vi "DatabaseHand_FindSubElement.vi"(8 "error in (no error)":errorcluster, 10 "name":string, 11 "Database RefNum in":T3) -> (0 "error out":errorcluster, 1 "index":i32, 2 "Database":T1, 3 "Database RefNum out":T3, 4 "object index":i32)   [LabVIEW 2016]
doc: "This VI finds the RefNum of an existing object with the input Name or creates a new object if the Name is not found or Name is unwired or an empty string.\nCopyright 2001 VI Engineering, Inc."
uses:
  DatabaseHand_RefNum.ctl
  DatabaseHand_Element.ctl
  DatabaseHan_DatabaseElement.ctl
  DatabaseHand_Function.ctl
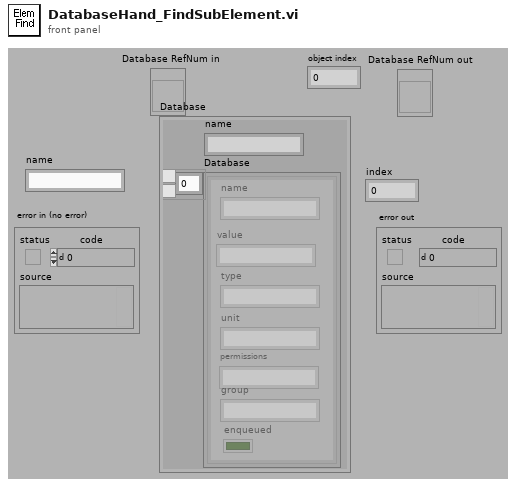
[diagram p1: front panel]
types:
  T1 = typedef "DatabaseHand_Element.ctl" = cluster{"name":string, "Database":T2[]}
  T2 = typedef "DatabaseHan_DatabaseElement.ctl" = cluster{"name":string, "value":string, "type":string, "unit":string, "permissions":string, "enqueued":bool, "group":string}
  T3 = typedef "DatabaseHand_RefNum.ctl" = refnum<vi>
  T4 = typedef "DatabaseHand_Function.ctl" = enum16{"Reset", "Register", "Get Data", "Set Data", "Unregister", "Test", "Get Objects", "Delete Data"}
  T5 = typedef "Database_Refnum.ctl" = refnum<vi>
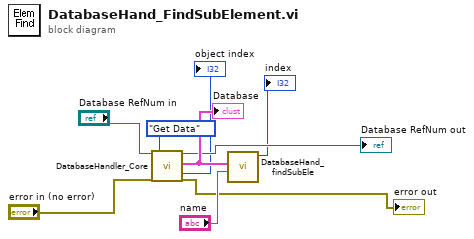
[diagram p0: block diagram]
diagram:
  n1 = call "DatabaseHandler_Core.vi"("Object Refnum In"="Database RefNum in", "error in (no error)"="error in (no error)", "Function (Get Data)"=DatabaseHand_Function."Get Data") -> ("Object Refnum out"=→"Database RefNum out":T5, "Object Data Out"=w6:T1, "object index"=→"object index":i32, "error out"=→"error out":errorcluster)  [unwired: 4 in, 9 out]
  "Database" <- w6
  n2 = call "DatabaseHand_findSubEle.vi"("name"="name", "Data In"=w6) -> ("index"=→"index":i32)  [unwired: 9 out]
